vi "Post-Build Action (App Dir True).vi"(5 "Files Generated by Build":path[](array[path]), 6 "Top Level/Always Included VIs":path[](array[path]), 7 "Destination Path":path, 8 "error in (no error)":errorcluster, 9 "Target Name":string, 10 "Build Specification Name":string, 11 "Project Path":path) -> (0 "error out":errorcluster)   [LabVIEW 2016]
uses:
  <vilib>/Utility/config.llb/Write Key (Boolean).vi
  <vilib>/Utility/config.llb/NI_LVConfig.lvlib
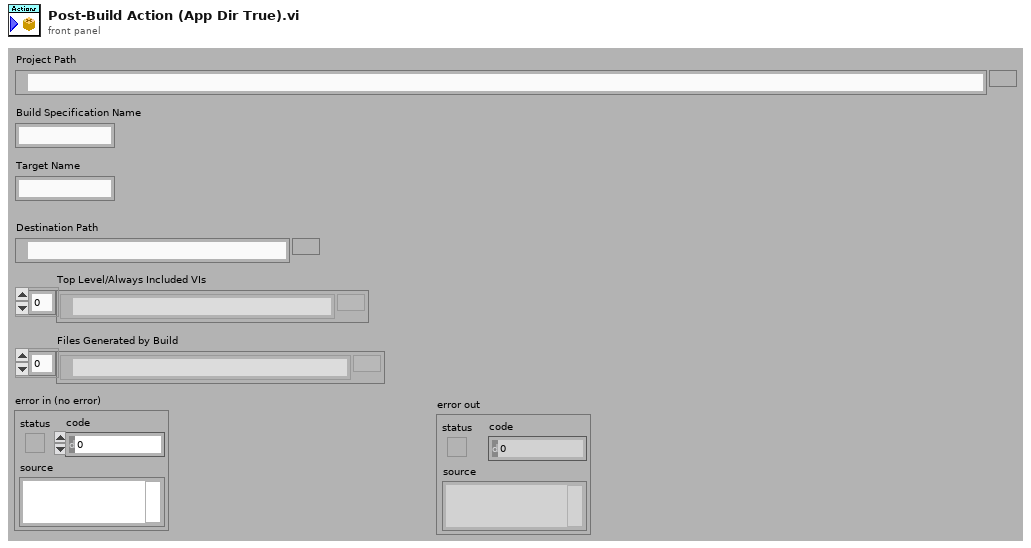
[diagram p1: front panel]
types:
  T1 = typedef "NI_LVConfig.lvlib/Config Data RefNum.ctl" = refnum<k1>
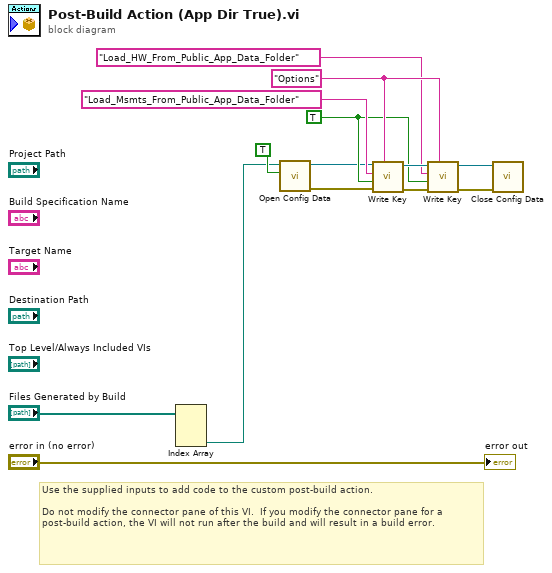
[diagram p0: block diagram]
diagram:
  w8 = TRUE ("value")
  w9 = "Options" ("section")
  # "Use the supplied inputs to add code to the custom post-build action.\n\nDo not modify the connector pane of this VI.  If you modify the connector pane for a post-build action, the VI will not run after the build and will result in a build error."
  n1 = Index Array(array="Files Generated by Build") -> (element #3=w2:path)  [unwired: 3 in, 2 out]
  n2 = call <vilib>:"Open Config Data.vi"("create file if necessary (T)"=TRUE, "configuration file path"=w2) -> ("error out"=w5:errorcluster, "refnum"=w6:T1)  [unwired: 7 in, 1 out]
  n3 = call-poly <vilib>:"Write Key.vi"("section"=w9, "error in (no error)"=w5, "value"=w8, "key"="Load_Msmts_From_Public_App_Data_Folder", "refnum"=w6) -> ("error out"=w12:errorcluster, "refnum out"=w11:T1)  [unwired: 4 in, 1 out]
  n4 = call-poly <vilib>:"Write Key.vi"("section"=w9, "error in (no error)"=w12, "value"=w8, "key"="Load_HW_From_Public_App_Data_Folder", "refnum"=w11) -> ("error out"=w4:errorcluster, "refnum out"=w3:T1)  [unwired: 4 in, 1 out]
  n5 = call <vilib>:"Close Config Data.vi"("error in (no error)"=w4, "refnum"=w3) -> ()  [unwired: 8 in, 2 out]
  "error out" <- "error in (no error)"
